vi "UDLR (Vectors).vi"() -> (3 "UDLR (Vectors)":cluster{"x":i16, "y":i16}[](array[cluster]))   [LabVIEW 2025, in "AOC.lvlib"]
uses:
  AOC.lvlib
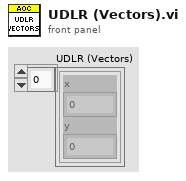
[diagram p1: front panel]
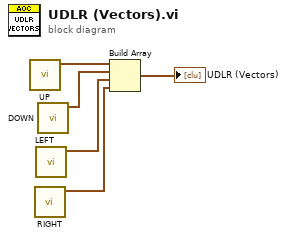
[diagram p0: block diagram]
diagram:
  n1 = call "UP.vi"() -> ("UP"=w1:cluster{"x":i16, "y":i16})  [unwired: 11 in]
  n2 = call "RIGHT.vi"() -> ("RIGHT"=w4:cluster{"x":i16, "y":i16})  [unwired: 11 in]
  n3 = call "LEFT.vi"() -> ("LEFT"=w3:cluster{"x":i16, "y":i16})  [unwired: 11 in]
  n4 = call "DOWN.vi"() -> ("DOWN"=w2:cluster{"x":i16, "y":i16})  [unwired: 11 in]
  n5 = Build Array(w1, w2, w3, w4) -> (→"UDLR (Vectors)":cluster{"x":i16, "y":i16}[])
